vi "Read VI Name.vi"(8 "error in (no error)":errorcluster, 11 "Tagbus PID Module configuration in":refnum<class "Tagbus PID Module configuration.lvclass">) -> (0 "error out":errorcluster, 2 "VI Name":string, 3 "Tagbus PID Module configuration out":refnum<class "Tagbus PID Module configuration.lvclass">)   [LabVIEW 2014]
uses:
  Tagbus PID Module configuration.lvclass
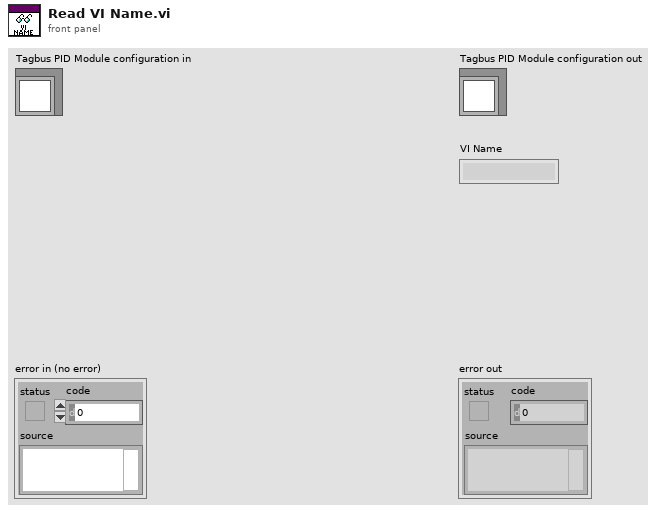
[diagram p1: front panel]
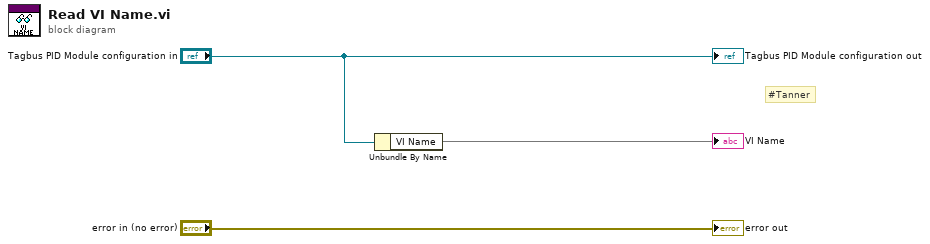
[diagram p0: block diagram]
diagram:
  # "#Tanner"
  n1 = Unbundle By Name("Tagbus PID Module configuration in") -> ("VI Name"=→"VI Name")
  "error out" <- "error in (no error)"
  "Tagbus PID Module configuration out" <- "Tagbus PID Module configuration in"
